vi "Main Targeting.vi"() -> ()   [LabVIEW 2013]
uses:
  <vilib>/Analysis/NI_AALPro.lvlib
panel:
  in  "Claw Angle":dbl[](array[numeric])
  in  "Distance":dbl[](array[numeric])
  out "Suggested Angle":dbl
  in  "Distance":dbl
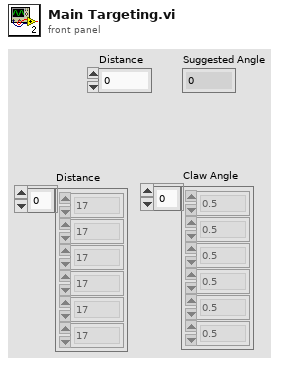
[diagram p1: front panel]
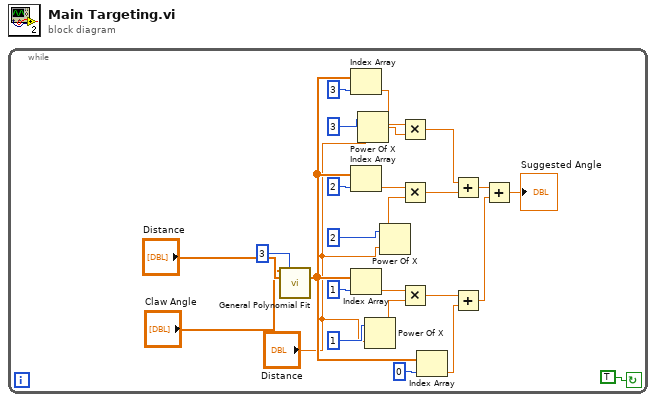
[diagram p0: block diagram]
diagram:
  n1 = while {
    stop <- TRUE continue-if-true
    n2 = call <vilib>:"General Polynomial Fit.vi"("Y"="Claw Angle", "polynomial order"=3, "X"="Distance") -> ("Polynomial Coefficients"=w16:dbl[])  [unwired: 9 in, 3 out]
    n3 = Index Array(array=w16, index=3) -> (element=w20:dbl)
    n4 = Index Array(array=w16, index=2) -> (element=w17:dbl)
    n5 = Index Array(array=w16, index=1) -> (element=w15:dbl)
    n6 = Power Of X(1:"Distance", 2:3) -> (0:w19:dbl)
    n7 = Power Of X(1:"Distance", 2:1) -> (0:w14:dbl)
    n8 = Power Of X(1:"Distance", 2:2) -> (0:w18:dbl)
    n9 = Multiply(x=w20, y=w19) -> (x*y=w13:dbl)
    n10 = Multiply(x=w17, y=w18) -> (x*y=w12:dbl)
    n11 = Multiply(x=w15, y=w14) -> (x*y=w10:dbl)
    n12 = Index Array(array=w16, index=0) -> (element=w11:dbl)
    n13 = Add(x=w13, y=w12) -> (x+y=w9:dbl)
    n14 = Add(x=w10, y=w11) -> (x+y=w8:dbl)
    n15 = Add(x=w9, y=w8) -> (x+y=→"Suggested Angle":dbl)
  }
